vi "Initialize Output DMA Refs.vi"(8 "error in (no error)":errorcluster, 10 "Settings.Compiled":T1 {"IncomingRegisters.Settings"."Register"."Data Type" format="%.0x"; "IncomingRegisters.Refs"."Refs"."Data Reference" format="%.0x"; "OutgoingRegisters.Settings"."Register"."Data Type" format="%.0x"; "OutgoingRegisters.Refs"."Refs"."Data Reference" format="%.0x"; "IncomingDMA.Settings"."Data Type" format="%.0x"; "IncomingDMA.Settings"."DMA.Settings"."DMA Host Buffer" items=["1 Second"=1, "2 Seconds"=2, "5 Seconds"=5, "10 Seconds"=10]; "IncomingDMA.Settings"."DMA.Settings"."dt" format="%#_p"; "IncomingDMA.Settings"."DMA.Settings"."Update Rate" items=["1 Hz"=1, "2 Hz"=2, "5 Hz"=5, "10 Hz"=10]; "OutgoingDMA.Settings"."Data Type" format="%.0x"; "OutgoingDMA.Settings"."DMA.Settings"."DMA Host Buffer" items=["1 Second"=1, "2 Seconds"=2, "5 Seconds"=5, "10 Seconds"=10]; "OutgoingDMA.Settings"."DMA.Settings"."dt" format="%#_p"; "OutgoingDMA.Settings"."DMA.Settings"."Update Rate" items=["1 Hz"=1, "2 Hz"=2, "5 Hz"=5, "10 Hz"=10]}, 11 "FPGA Ref":refnum<k20>) -> (0 "error out":errorcluster, 2 "DMA":T15[](array[typedef]) {"Refs"."Data Type" format="%.0x"}, 3 "FPGA Ref":refnum<k20>)   [LabVIEW 2024, in "FPGA Addon Engine.lvlib"]
uses:
  FPGA Addon Engine.lvlib
  Types/DMA Output References.ctl
  <vilib>/NI VeriStand/Custom Device Waveform API/Single Waveform Read (DBL)/Single Waveform Read (DBL).lvclass
  Types/DMA Output Refs.ctl
  Addon Shared/Types/FPGA Addon Data Type.ctl
  Addon Shared/Types/Compiled.Settings.ctl
  Addon Shared/Types/Compiled.RegisterSettings.ctl
  Addon Shared/Types/Scalar Type.ctl
  Addon Shared/Types/Register Information.ctl
  <vilib>/NI VeriStand/Custom Device API/Block Data Reference.ctl
  <vilib>/NI VeriStand/Custom Device API/Data Reference.ctl
  Addon Shared/Types/Compiled.DMASettings.ctl
  Addon Shared/Types/DMA Settings.ctl
  Addon Shared/Types/Delacing Scheme.ctl
  Addon Shared/Types/DMA Acquisition Mode.ctl
  <vilib>/NI VeriStand/Custom Device API/Waveform Data Reference.ctl
  Addon Shared/Types/FPGA Settings.ctl
  <vilib>/NI VeriStand/Custom Device API/Custom Device Target Type.ctl
  <vilib>/NI/LVFPGA Adv Session Resources/OpenByNameSubVI.vi
  <vilib>/rvi/interface/common/dynamic/niFpgaEscapeDelimiterAndNull.vi
  <vilib>/Utility/error.llb/Error Cluster From Error Code.vi
  <vilib>/rvi/interface/common/niFpgaWaitOnOcc.vi
  <vilib>/NI VeriStand/Custom Device Waveform API/Single Waveform Read (DBL)/NI VeriStand - Open Single Waveform Read Session (DBL).vi
  <vilib>/NI/LVFPGA Adv Session Resources/OpenByName.xnode
  <vilib>/rvi/interface/nirviMethod/nirviMethod.xnode
  <vilib>/NI VeriStand/Custom Device Waveform API/NI_VS Custom Device Waveform API.lvlib
  <vilib>/rvi/errors/niLvFpgaMergeErrorWithErrorCode.vi
  <vilib>/FPGAPlugInAG/Dynamic/niLvFpga_ConfigureFifo_Dynamic.vi
  <vilib>/FPGAPlugInAG/Dynamic/niLvFpga_StartFifo_Dynamic.vi
  <vilib>/NI/LVFPGA Adv Session Resources/LVFPGAAdvSessionResources.lvlib
  Addon Shared/FPGA Addon Shared.lvlib
  <vilib>/NI VeriStand/Custom Device API/Custom Device API.lvlib
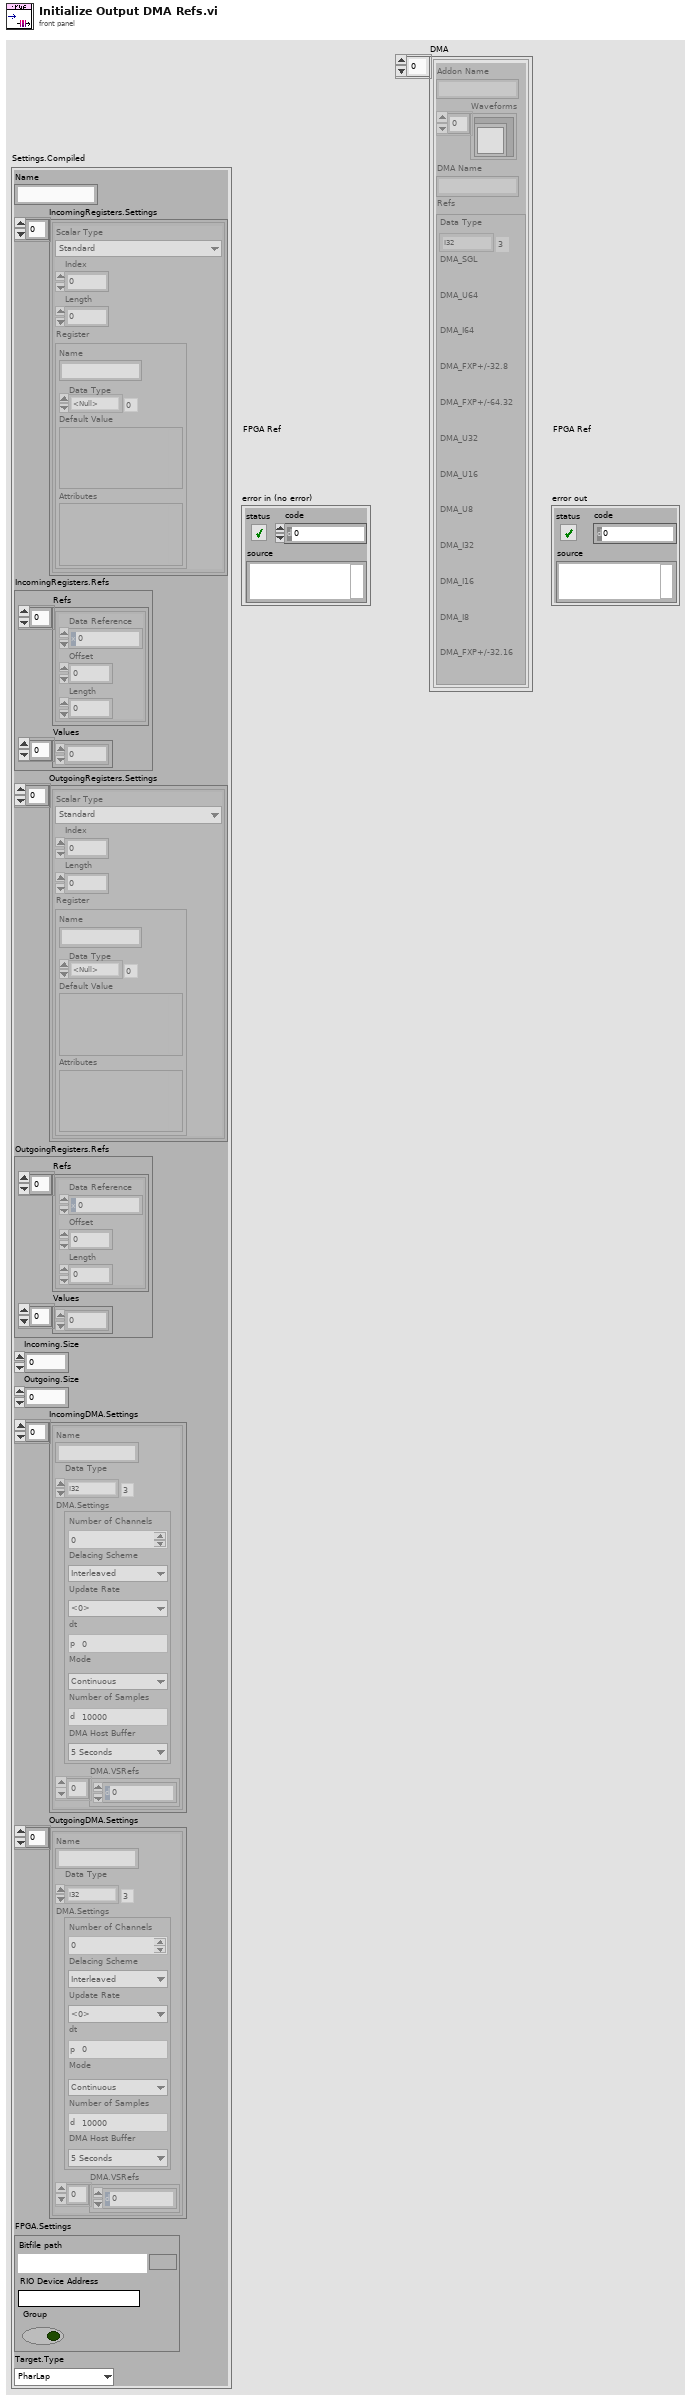
[diagram p1: front panel]
types:
  T1 = typedef "FPGA Addon Shared.lvlib/Compiled.Settings.ctl" = cluster{"Name":string, "IncomingRegisters.Settings":T2[], "IncomingRegisters.Refs":cluster{"Refs":T6[], "Values":dbl[]}, "OutgoingRegisters.Settings":T2[], "OutgoingRegisters.Refs":cluster{"Refs":T6[], "Values":dbl[]}, "Incoming.Size":i32, "Outgoing.Size":i32, "IncomingDMA.Settings":T8[], "OutgoingDMA.Settings":T8[], "FPGA.Settings":T13, "Target.Type":T14}
  T2 = typedef "FPGA Addon Shared.lvlib/Compiled.RegisterSettings.ctl" = cluster{"Scalar Type":T3, "Index":i32, "Length":i32, "Register":T4}
  T3 = typedef "FPGA Addon Shared.lvlib/Scalar Type.ctl" = enum16{"Standard", "Bitpacked"}
  T4 = typedef "FPGA Addon Shared.lvlib/Register Information.ctl" = cluster{"Name":string, "Data Type":T5, "Default Value":variant, "Attributes":variant}
  T5 = typedef "FPGA Addon Shared.lvlib/FPGA Addon Data Type.ctl" = enum8{"<Null>", "I8", "I16", "I32", "I64", "U8", "U16", "U32", "U64", "SGL", "Boolean", "Analog PWM In Settings", "Analog PWM In", "Digital PWM In Settings", "Digital PWM In", "Digital PWM Out", "Sine Out", "FXP", "FXP+/-24.5", "FXP+/-16.5", "FXP+/-32.8", "FXP+/-64.32", "FXP+/-16.7", "FXP+/-20.5", "FXP+/-27.5", "FXP+/-32.16", "FXP+16.3", "FXP+18.3", "Digital Static In", "Digital Static Out", "Digital Static In Settings", "Digital WSS Out", "Quad Encoder Settings", "Quad Encoder In", "Group"}
  T6 = typedef "Custom Device API.lvlib/Block Data Reference.ctl" = cluster{"Data Reference":T7, "Offset":u64, "Length":u64}
  T7 = typedef "Custom Device API.lvlib/Data Reference.ctl" = i32
  T8 = typedef "FPGA Addon Shared.lvlib/Compiled.DMASettings.ctl" = cluster{"Name":string, "Data Type":T5, "DMA.Settings":T9, "DMA.VSRefs":T12[]}
  T9 = typedef "FPGA Addon Shared.lvlib/DMA Settings.ctl" = cluster{"Number of Channels":u8, "Delacing Scheme":T10, "Update Rate":u32, "dt":dbl, "Mode":T11, "Number of Samples":u32, "DMA Host Buffer":u32}
  T10 = typedef "FPGA Addon Shared.lvlib/Delacing Scheme.ctl" = enum8{"Interleaved", "Bitpacked"}
  T11 = typedef "FPGA Addon Shared.lvlib/DMA Acquisition Mode.ctl" = enum8{"Continuous", "Triggered Finite"}
  T12 = typedef "Custom Device API.lvlib/Waveform Data Reference.ctl" = i32
  T13 = typedef "FPGA Addon Shared.lvlib/FPGA Settings.ctl" = cluster{"Bitfile path":path, "RIO Device Address":string, "Group":bool}
  T14 = typedef "Custom Device API.lvlib/Custom Device Target Type.ctl" = enum16{"PharLap", "VxWorks", "Windows", "Linux_32_ARM", "Linux_x64"}
  T15 = typedef "FPGA Addon Engine.lvlib/DMA Output References.ctl" = cluster{"Addon Name":string, "Waveforms":refnum<class "Single Waveform Read (DBL).lvclass">[], "DMA Name":string, "Refs":T16}
  T16 = typedef "FPGA Addon Engine.lvlib/DMA Output Refs.ctl" = cluster{"Data Type":T5, "DMA_SGL":refnum<k20>, "DMA_U64":refnum<k20>, "DMA_I64":refnum<k20>, "DMA_FXP+/-32.8":refnum<k20>, "DMA_FXP+/-64.32":refnum<k20>, "DMA_U32":refnum<k20>, "DMA_U16":refnum<k20>, "DMA_U8":refnum<k20>, "DMA_I32":refnum<k20>, "DMA_I16":refnum<k20>, "DMA_I8":refnum<k20>, "DMA_FXP+/-32.16":refnum<k20>}
  T17 = cluster{"Name":string, "Depth":u32, "Write? (Deprecated:Use Implementation)":bool, "Physical Channel":u32, "Base Address":u32, "Data Width":u32, "Data Type":enum32{"Boolean", "I8", "I16", "I32", "I64", "U8", "U16", "U32", "U64", "FXP", "CustomControl", "SGL"}, "FXP Properties":variant, "Write Window Address":u32, "Implementation":enum16{"niFpgaTargetToHost", "niFpgaHostToTarget", "niFpgaPeerToPeerWriter", "niFpgaPeerToPeerReader", "niCoreTargetToHost", "niCoreHostToTarget"}, "Control Set":u32}[]
  T18 = cluster{"Name":string, "type":variant, "indicator?":bool}[]
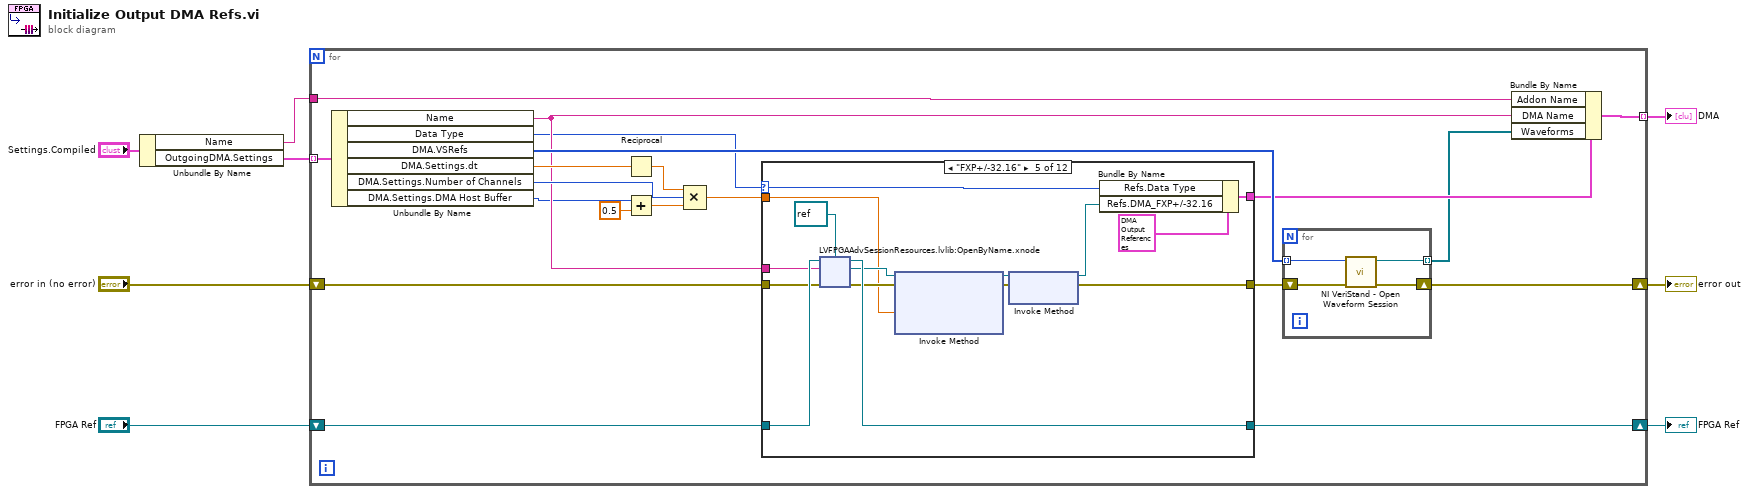
[diagram p0: block diagram]
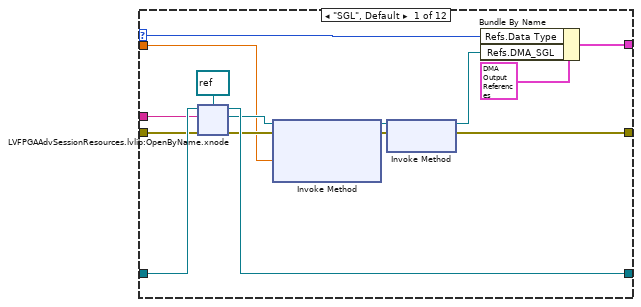
[diagram p2: hidden frame]
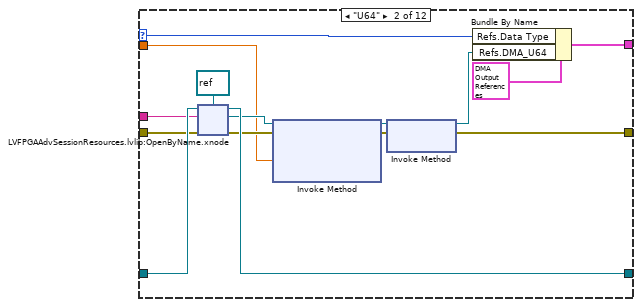
[diagram p3: hidden frame]
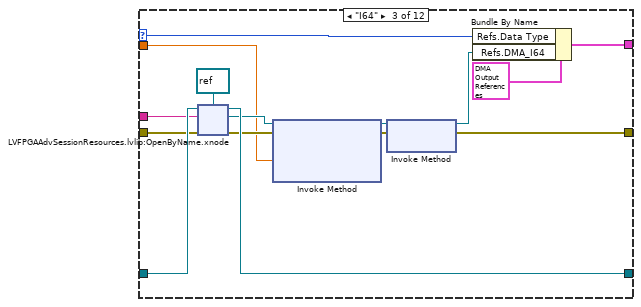
[diagram p4: hidden frame]
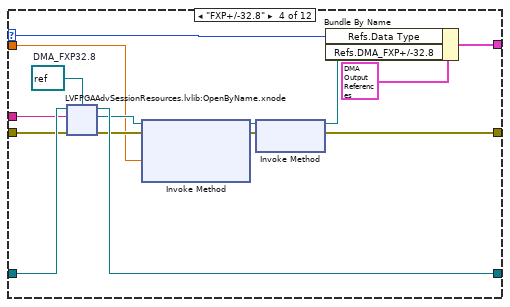
[diagram p5: hidden frame]
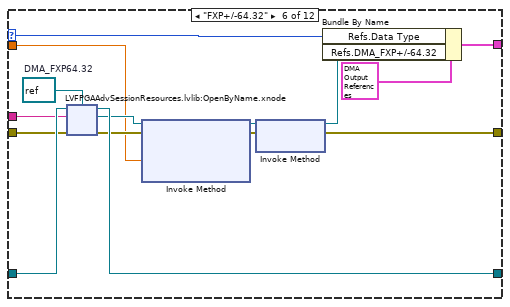
[diagram p6: hidden frame]
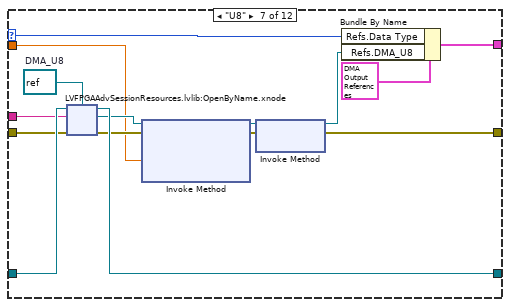
[diagram p7: hidden frame]
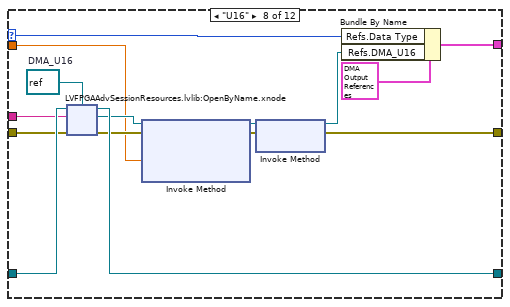
[diagram p8: hidden frame]
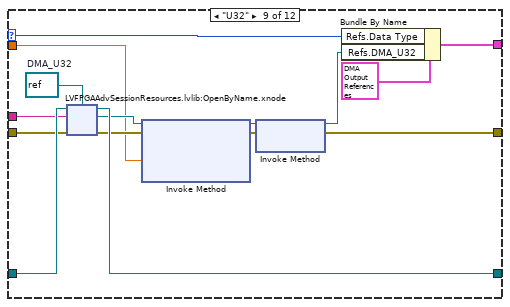
[diagram p9: hidden frame]
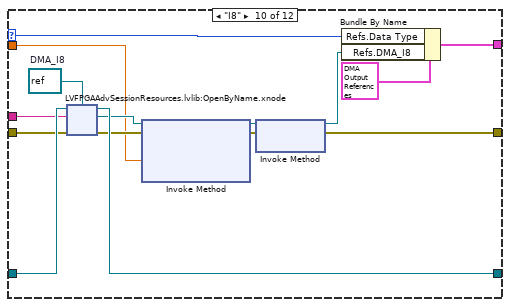
[diagram p10: hidden frame]
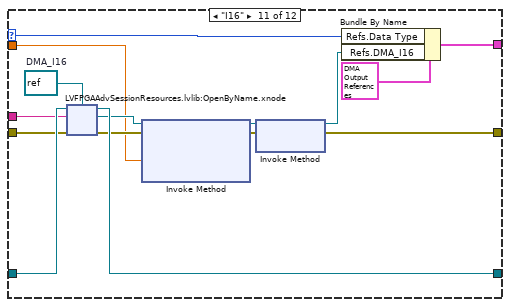
[diagram p11: hidden frame]
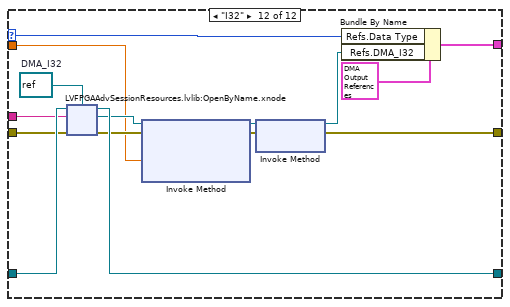
[diagram p12: hidden frame]
diagram:
  n1 = Unbundle By Name("Settings.Compiled") -> ("Name"=w1:string, "OutgoingDMA.Settings"=w3:T8[])
  n2 = for {
    shift-right: [w17] -> w6
    shift-left: "error in (no error)" -> [w22]
    shift-right: [w27] -> w7
    shift-left: "FPGA Ref" -> [w28]
    tunnel: [w26] -> w5 mode=indexing
    tunnel: w3 -> [w24] mode=indexing
    tunnel: w1 -> [w9]
    n3 = Unbundle By Name(w24) -> ("Name"=w19:string, "Data Type"=w10:T5, "DMA.VSRefs"=w23:T12[], "DMA.Settings.dt"=w21:dbl, "DMA.Settings.Number of Channels"=w20:u8, "DMA.Settings.DMA Host Buffer"=w15:u32)
    n4 = Reciprocal(x=w21) -> (1/x=w16:dbl)
    n5 = Add(x=w15, y=0.5) -> (x+y=w14:dbl)
    n6 = Compound Arithmetic op=MULTIPLY(w16, w20, w14) -> (w25:dbl)
    n7 = case shown="\"FXP+/-32.16\"" w10 {
      selector: w10 -> [w29 w57 w86 w114 w143 w170 w198 w226 w254 w282 w310 w338]
      tunnel: w28 -> [w42 w71 w99 w127 w155 w183 w211 w239 w267 w295 w323 w351]
      tunnel: [w41 w70 w98 w126 w154 w182 w210 w238 w266 w294 w322 w350] -> w27
      tunnel: w25 -> [w35 w64 w92 w120 w148 w176 w204 w232 w260 w288 w316 w344]
      tunnel: w22 -> [w34 w63 w91 w119 w147 w175 w203 w231 w259 w287 w315 w343]
      tunnel: w19 -> [w33 w62 w90 w118 w146 w174 w202 w230 w258 w286 w314 w342]
      tunnel: [w32 w61 w89 w117 w145 w173 w201 w229 w257 w285 w313 w341] -> w18
      tunnel: [w31 w60 w88 w116 w144 w172 w200 w228 w256 w284 w312 w340] -> w12
      frame "SGL", Default {
        n8 = xnode "LVFPGAAdvSessionResources.lvlib:OpenByName.xnode"("FPGA VI Reference in"=w42, "Resource name in"=w33, "Single resource reference type in"=refnum<k20> refnum, "Error in"=w34) -> ("Single resource reference out"=w36:refnum<k20>, "Error out"=w37:errorcluster, "FPGA VI Reference out"=w41:refnum<k20>)
        n9 = xnode "Invoke Method"("FPGA VI Reference In"=w36, "error in"=w37, "Requested Depth"=w35) -> ("FPGA VI Reference Out"=w39:refnum<k20>, "error out"=w38:errorcluster)  [unwired: 1 out]
        n10 = xnode "Invoke Method"("FPGA VI Reference In"=w39, "error in"=w38) -> ("FPGA VI Reference Out"=w30:refnum<k20>, "error out"=w32:errorcluster)
        n11 = Bundle By Name(cluster=T15 {"Addon Name"="", "Waveforms"=[], "DMA Name"="", "Refs"={"Data Type"=enum."I32", "DMA_SGL"=refnum, "DMA_U64"=refnum, "DMA_I64"=refnum, "DMA_FXP+/-32.8"=refnum, "DMA_FXP+/-64.32"=refnum, "DMA_U32"=refnum, "DMA_U16"=refnum, "DMA_U8"=refnum, "DMA_I32"=refnum, "DMA_I16"=refnum, "DMA_I8"=refnum, "DMA_FXP+/-32.16"=refnum}}, "Refs.Data Type"=w29, "Refs.DMA_SGL"=w30) -> (w31:T15)
      }
      frame "U64" {
        n12 = xnode "LVFPGAAdvSessionResources.lvlib:OpenByName.xnode"("FPGA VI Reference in"=w71, "Resource name in"=w62, "Single resource reference type in"=refnum<k20> refnum ("DMA_U64"), "Error in"=w63) -> ("Single resource reference out"=w65:refnum<k20>, "Error out"=w66:errorcluster, "FPGA VI Reference out"=w70:refnum<k20>)
        n13 = xnode "Invoke Method"("FPGA VI Reference In"=w65, "error in"=w66, "Requested Depth"=w64) -> ("FPGA VI Reference Out"=w68:refnum<k20>, "error out"=w67:errorcluster)  [unwired: 1 out]
        n14 = xnode "Invoke Method"("FPGA VI Reference In"=w68, "error in"=w67) -> ("FPGA VI Reference Out"=w59:refnum<k20>, "error out"=w61:errorcluster)
        n15 = Bundle By Name(cluster=T15 {"Addon Name"="", "Waveforms"=[], "DMA Name"="", "Refs"={"Data Type"=enum."I32", "DMA_SGL"=refnum, "DMA_U64"=refnum, "DMA_I64"=refnum, "DMA_FXP+/-32.8"=refnum, "DMA_FXP+/-64.32"=refnum, "DMA_U32"=refnum, "DMA_U16"=refnum, "DMA_U8"=refnum, "DMA_I32"=refnum, "DMA_I16"=refnum, "DMA_I8"=refnum, "DMA_FXP+/-32.16"=refnum}}, "Refs.Data Type"=w57, "Refs.DMA_U64"=w59) -> (w60:T15)
      }
      frame "I64" {
        n16 = xnode "LVFPGAAdvSessionResources.lvlib:OpenByName.xnode"("FPGA VI Reference in"=w99, "Resource name in"=w90, "Single resource reference type in"=refnum<k20> refnum ("DMA_I64"), "Error in"=w91) -> ("Single resource reference out"=w93:refnum<k20>, "Error out"=w94:errorcluster, "FPGA VI Reference out"=w98:refnum<k20>)
        n17 = xnode "Invoke Method"("FPGA VI Reference In"=w93, "error in"=w94, "Requested Depth"=w92) -> ("FPGA VI Reference Out"=w96:refnum<k20>, "error out"=w95:errorcluster)  [unwired: 1 out]
        n18 = xnode "Invoke Method"("FPGA VI Reference In"=w96, "error in"=w95) -> ("FPGA VI Reference Out"=w87:refnum<k20>, "error out"=w89:errorcluster)
        n19 = Bundle By Name(cluster=T15 {"Addon Name"="", "Waveforms"=[], "DMA Name"="", "Refs"={"Data Type"=enum."I32", "DMA_SGL"=refnum, "DMA_U64"=refnum, "DMA_I64"=refnum, "DMA_FXP+/-32.8"=refnum, "DMA_FXP+/-64.32"=refnum, "DMA_U32"=refnum, "DMA_U16"=refnum, "DMA_U8"=refnum, "DMA_I32"=refnum, "DMA_I16"=refnum, "DMA_I8"=refnum, "DMA_FXP+/-32.16"=refnum}}, "Refs.Data Type"=w86, "Refs.DMA_I64"=w87) -> (w88:T15)
      }
      frame "FXP+/-32.8" {
        w113 = refnum<k20> refnum  # DMA_FXP32.8
        n20 = xnode "LVFPGAAdvSessionResources.lvlib:OpenByName.xnode"("FPGA VI Reference in"=w127, "Resource name in"=w118, "Single resource reference type in"=w113, "Error in"=w119) -> ("Single resource reference out"=w121:refnum<k20>, "Error out"=w122:errorcluster, "FPGA VI Reference out"=w126:refnum<k20>)
        n21 = xnode "Invoke Method"("FPGA VI Reference In"=w121, "error in"=w122, "Requested Depth"=w120) -> ("FPGA VI Reference Out"=w124:refnum<k20>, "error out"=w123:errorcluster)  [unwired: 1 out]
        n22 = xnode "Invoke Method"("FPGA VI Reference In"=w124, "error in"=w123) -> ("FPGA VI Reference Out"=w115:refnum<k20>, "error out"=w117:errorcluster)
        n23 = Bundle By Name(cluster=T15 {"Addon Name"="", "Waveforms"=[], "DMA Name"="", "Refs"={"Data Type"=enum."I32", "DMA_SGL"=refnum, "DMA_U64"=refnum, "DMA_I64"=refnum, "DMA_FXP+/-32.8"=refnum, "DMA_FXP+/-64.32"=refnum, "DMA_U32"=refnum, "DMA_U16"=refnum, "DMA_U8"=refnum, "DMA_I32"=refnum, "DMA_I16"=refnum, "DMA_I8"=refnum, "DMA_FXP+/-32.16"=refnum}}, "Refs.Data Type"=w114, "Refs.DMA_FXP+/-32.8"=w115) -> (w116:T15)
      }
      frame "FXP+/-32.16" {
        n24 = xnode "LVFPGAAdvSessionResources.lvlib:OpenByName.xnode"("FPGA VI Reference in"=w155, "Resource name in"=w146, "Single resource reference type in"=refnum<k20> refnum ("Refs.DMA_FXP+/-32.16"), "Error in"=w147) -> ("Single resource reference out"=w149:refnum<k20>, "Error out"=w150:errorcluster, "FPGA VI Reference out"=w154:refnum<k20>)
        n25 = xnode "Invoke Method"("FPGA VI Reference In"=w149, "error in"=w150, "Requested Depth"=w148) -> ("FPGA VI Reference Out"=w152:refnum<k20>, "error out"=w151:errorcluster)  [unwired: 1 out]
        n26 = xnode "Invoke Method"("FPGA VI Reference In"=w152, "error in"=w151) -> ("FPGA VI Reference Out"=w141:refnum<k20>, "error out"=w145:errorcluster)
        n27 = Bundle By Name(cluster=T15 {"Addon Name"="", "Waveforms"=[], "DMA Name"="", "Refs"={"Data Type"=enum."I32", "DMA_SGL"=refnum, "DMA_U64"=refnum, "DMA_I64"=refnum, "DMA_FXP+/-32.8"=refnum, "DMA_FXP+/-64.32"=refnum, "DMA_U32"=refnum, "DMA_U16"=refnum, "DMA_U8"=refnum, "DMA_I32"=refnum, "DMA_I16"=refnum, "DMA_I8"=refnum, "DMA_FXP+/-32.16"=refnum}}, "Refs.Data Type"=w143, "Refs.DMA_FXP+/-32.16"=w141) -> (w144:T15)
      }
      frame "FXP+/-64.32" {
        w169 = refnum<k20> refnum  # DMA_FXP64.32
        n28 = xnode "LVFPGAAdvSessionResources.lvlib:OpenByName.xnode"("FPGA VI Reference in"=w183, "Resource name in"=w174, "Single resource reference type in"=w169, "Error in"=w175) -> ("Single resource reference out"=w177:refnum<k20>, "Error out"=w178:errorcluster, "FPGA VI Reference out"=w182:refnum<k20>)
        n29 = xnode "Invoke Method"("FPGA VI Reference In"=w177, "error in"=w178, "Requested Depth"=w176) -> ("FPGA VI Reference Out"=w180:refnum<k20>, "error out"=w179:errorcluster)  [unwired: 1 out]
        n30 = xnode "Invoke Method"("FPGA VI Reference In"=w180, "error in"=w179) -> ("FPGA VI Reference Out"=w171:refnum<k20>, "error out"=w173:errorcluster)
        n31 = Bundle By Name(cluster=T15 {"Addon Name"="", "Waveforms"=[], "DMA Name"="", "Refs"={"Data Type"=enum."I32", "DMA_SGL"=refnum, "DMA_U64"=refnum, "DMA_I64"=refnum, "DMA_FXP+/-32.8"=refnum, "DMA_FXP+/-64.32"=refnum, "DMA_U32"=refnum, "DMA_U16"=refnum, "DMA_U8"=refnum, "DMA_I32"=refnum, "DMA_I16"=refnum, "DMA_I8"=refnum, "DMA_FXP+/-32.16"=refnum}}, "Refs.Data Type"=w170, "Refs.DMA_FXP+/-64.32"=w171) -> (w172:T15)
      }
      frame "U8" {
        w197 = refnum<k20> refnum  # DMA_U8
        n32 = xnode "LVFPGAAdvSessionResources.lvlib:OpenByName.xnode"("FPGA VI Reference in"=w211, "Resource name in"=w202, "Single resource reference type in"=w197, "Error in"=w203) -> ("Single resource reference out"=w205:refnum<k20>, "Error out"=w206:errorcluster, "FPGA VI Reference out"=w210:refnum<k20>)
        n33 = xnode "Invoke Method"("FPGA VI Reference In"=w205, "error in"=w206, "Requested Depth"=w204) -> ("FPGA VI Reference Out"=w208:refnum<k20>, "error out"=w207:errorcluster)  [unwired: 1 out]
        n34 = xnode "Invoke Method"("FPGA VI Reference In"=w208, "error in"=w207) -> ("FPGA VI Reference Out"=w199:refnum<k20>, "error out"=w201:errorcluster)
        n35 = Bundle By Name(cluster=T15 {"Addon Name"="", "Waveforms"=[], "DMA Name"="", "Refs"={"Data Type"=enum."I32", "DMA_SGL"=refnum, "DMA_U64"=refnum, "DMA_I64"=refnum, "DMA_FXP+/-32.8"=refnum, "DMA_FXP+/-64.32"=refnum, "DMA_U32"=refnum, "DMA_U16"=refnum, "DMA_U8"=refnum, "DMA_I32"=refnum, "DMA_I16"=refnum, "DMA_I8"=refnum, "DMA_FXP+/-32.16"=refnum}}, "Refs.Data Type"=w198, "Refs.DMA_U8"=w199) -> (w200:T15)
      }
      frame "U16" {
        w225 = refnum<k20> refnum  # DMA_U16
        n36 = xnode "LVFPGAAdvSessionResources.lvlib:OpenByName.xnode"("FPGA VI Reference in"=w239, "Resource name in"=w230, "Single resource reference type in"=w225, "Error in"=w231) -> ("Single resource reference out"=w233:refnum<k20>, "Error out"=w234:errorcluster, "FPGA VI Reference out"=w238:refnum<k20>)
        n37 = xnode "Invoke Method"("FPGA VI Reference In"=w233, "error in"=w234, "Requested Depth"=w232) -> ("FPGA VI Reference Out"=w236:refnum<k20>, "error out"=w235:errorcluster)  [unwired: 1 out]
        n38 = xnode "Invoke Method"("FPGA VI Reference In"=w236, "error in"=w235) -> ("FPGA VI Reference Out"=w227:refnum<k20>, "error out"=w229:errorcluster)
        n39 = Bundle By Name(cluster=T15 {"Addon Name"="", "Waveforms"=[], "DMA Name"="", "Refs"={"Data Type"=enum."I32", "DMA_SGL"=refnum, "DMA_U64"=refnum, "DMA_I64"=refnum, "DMA_FXP+/-32.8"=refnum, "DMA_FXP+/-64.32"=refnum, "DMA_U32"=refnum, "DMA_U16"=refnum, "DMA_U8"=refnum, "DMA_I32"=refnum, "DMA_I16"=refnum, "DMA_I8"=refnum, "DMA_FXP+/-32.16"=refnum}}, "Refs.Data Type"=w226, "Refs.DMA_U16"=w227) -> (w228:T15)
      }
      frame "U32" {
        w253 = refnum<k20> refnum  # DMA_U32
        n40 = xnode "LVFPGAAdvSessionResources.lvlib:OpenByName.xnode"("FPGA VI Reference in"=w267, "Resource name in"=w258, "Single resource reference type in"=w253, "Error in"=w259) -> ("Single resource reference out"=w261:refnum<k20>, "Error out"=w262:errorcluster, "FPGA VI Reference out"=w266:refnum<k20>)
        n41 = xnode "Invoke Method"("FPGA VI Reference In"=w261, "error in"=w262, "Requested Depth"=w260) -> ("FPGA VI Reference Out"=w264:refnum<k20>, "error out"=w263:errorcluster)  [unwired: 1 out]
        n42 = xnode "Invoke Method"("FPGA VI Reference In"=w264, "error in"=w263) -> ("FPGA VI Reference Out"=w255:refnum<k20>, "error out"=w257:errorcluster)
        n43 = Bundle By Name(cluster=T15 {"Addon Name"="", "Waveforms"=[], "DMA Name"="", "Refs"={"Data Type"=enum."I32", "DMA_SGL"=refnum, "DMA_U64"=refnum, "DMA_I64"=refnum, "DMA_FXP+/-32.8"=refnum, "DMA_FXP+/-64.32"=refnum, "DMA_U32"=refnum, "DMA_U16"=refnum, "DMA_U8"=refnum, "DMA_I32"=refnum, "DMA_I16"=refnum, "DMA_I8"=refnum, "DMA_FXP+/-32.16"=refnum}}, "Refs.Data Type"=w254, "Refs.DMA_U32"=w255) -> (w256:T15)
      }
      frame "I8" {
        w281 = refnum<k20> refnum  # DMA_I8
        n44 = xnode "LVFPGAAdvSessionResources.lvlib:OpenByName.xnode"("FPGA VI Reference in"=w295, "Resource name in"=w286, "Single resource reference type in"=w281, "Error in"=w287) -> ("Single resource reference out"=w289:refnum<k20>, "Error out"=w290:errorcluster, "FPGA VI Reference out"=w294:refnum<k20>)
        n45 = xnode "Invoke Method"("FPGA VI Reference In"=w289, "error in"=w290, "Requested Depth"=w288) -> ("FPGA VI Reference Out"=w292:refnum<k20>, "error out"=w291:errorcluster)  [unwired: 1 out]
        n46 = xnode "Invoke Method"("FPGA VI Reference In"=w292, "error in"=w291) -> ("FPGA VI Reference Out"=w283:refnum<k20>, "error out"=w285:errorcluster)
        n47 = Bundle By Name(cluster=T15 {"Addon Name"="", "Waveforms"=[], "DMA Name"="", "Refs"={"Data Type"=enum."I32", "DMA_SGL"=refnum, "DMA_U64"=refnum, "DMA_I64"=refnum, "DMA_FXP+/-32.8"=refnum, "DMA_FXP+/-64.32"=refnum, "DMA_U32"=refnum, "DMA_U16"=refnum, "DMA_U8"=refnum, "DMA_I32"=refnum, "DMA_I16"=refnum, "DMA_I8"=refnum, "DMA_FXP+/-32.16"=refnum}}, "Refs.Data Type"=w282, "Refs.DMA_I8"=w283) -> (w284:T15)
      }
      frame "I16" {
        w309 = refnum<k20> refnum  # DMA_I16
        n48 = xnode "LVFPGAAdvSessionResources.lvlib:OpenByName.xnode"("FPGA VI Reference in"=w323, "Resource name in"=w314, "Single resource reference type in"=w309, "Error in"=w315) -> ("Single resource reference out"=w317:refnum<k20>, "Error out"=w318:errorcluster, "FPGA VI Reference out"=w322:refnum<k20>)
        n49 = xnode "Invoke Method"("FPGA VI Reference In"=w317, "error in"=w318, "Requested Depth"=w316) -> ("FPGA VI Reference Out"=w320:refnum<k20>, "error out"=w319:errorcluster)  [unwired: 1 out]
        n50 = xnode "Invoke Method"("FPGA VI Reference In"=w320, "error in"=w319) -> ("FPGA VI Reference Out"=w311:refnum<k20>, "error out"=w313:errorcluster)
        n51 = Bundle By Name(cluster=T15 {"Addon Name"="", "Waveforms"=[], "DMA Name"="", "Refs"={"Data Type"=enum."I32", "DMA_SGL"=refnum, "DMA_U64"=refnum, "DMA_I64"=refnum, "DMA_FXP+/-32.8"=refnum, "DMA_FXP+/-64.32"=refnum, "DMA_U32"=refnum, "DMA_U16"=refnum, "DMA_U8"=refnum, "DMA_I32"=refnum, "DMA_I16"=refnum, "DMA_I8"=refnum, "DMA_FXP+/-32.16"=refnum}}, "Refs.Data Type"=w310, "Refs.DMA_I16"=w311) -> (w312:T15)
      }
      frame "I32" {
        w337 = refnum<k20> refnum  # DMA_I32
        n52 = xnode "LVFPGAAdvSessionResources.lvlib:OpenByName.xnode"("FPGA VI Reference in"=w351, "Resource name in"=w342, "Single resource reference type in"=w337, "Error in"=w343) -> ("Single resource reference out"=w345:refnum<k20>, "Error out"=w346:errorcluster, "FPGA VI Reference out"=w350:refnum<k20>)
        n53 = xnode "Invoke Method"("FPGA VI Reference In"=w345, "error in"=w346, "Requested Depth"=w344) -> ("FPGA VI Reference Out"=w348:refnum<k20>, "error out"=w347:errorcluster)  [unwired: 1 out]
        n54 = xnode "Invoke Method"("FPGA VI Reference In"=w348, "error in"=w347) -> ("FPGA VI Reference Out"=w339:refnum<k20>, "error out"=w341:errorcluster)
        n55 = Bundle By Name(cluster=T15 {"Addon Name"="", "Waveforms"=[], "DMA Name"="", "Refs"={"Data Type"=enum."I32", "DMA_SGL"=refnum, "DMA_U64"=refnum, "DMA_I64"=refnum, "DMA_FXP+/-32.8"=refnum, "DMA_FXP+/-64.32"=refnum, "DMA_U32"=refnum, "DMA_U16"=refnum, "DMA_U8"=refnum, "DMA_I32"=refnum, "DMA_I16"=refnum, "DMA_I8"=refnum, "DMA_FXP+/-32.16"=refnum}}, "Refs.Data Type"=w338, "Refs.DMA_I32"=w339) -> (w340:T15)
      }
    }
    n56 = for {
      shift-right: [w368] -> w17
      shift-left: w18 -> [w366]
      tunnel: [w367] -> w11 mode=indexing
      tunnel: w23 -> [w365] mode=indexing
      n57 = call-poly <vilib>:"NI VeriStand - Open Waveform Session.vi"("error in (no error)"=w366, "DBL Waveform Data Reference"=w365) -> ("error out"=w368:errorcluster, "Single Waveform Read Session (DBL)"=w367:refnum<class "Single Waveform Read (DBL).lvclass">)  [unwired: 8 in]
    }
    n58 = Bundle By Name(cluster=w12, "Addon Name"=w9, "DMA Name"=w19, "Waveforms"=w11) -> (w26:T15)
  }
  "error out" <- w6
  "FPGA Ref" <- w7
  "DMA" <- w5
